vi "FibreSqeezerVI.vi"() -> ()   [LabVIEW 2011]
uses:
  <vilib>/DAQmx/write.llb/DAQmx Write (Analog DBL 1Chan 1Samp).vi
  <vilib>/DAQmx/create/channels.llb/DAQmx Create Channel (AO-Voltage-Basic).vi
  <vilib>/DAQmx/configure/timing.llb/DAQmx Timing (Sample Clock).vi
  <vilib>/DAQmx/miscellaneous.llb/DAQmx Fill In Error Info.vi
  <vilib>/measure/NI_MABase.lvlib
panel:
  in  "frequency":dbl=10.0 format="%0.2p"
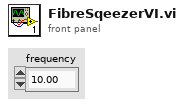
[diagram p1: front panel]
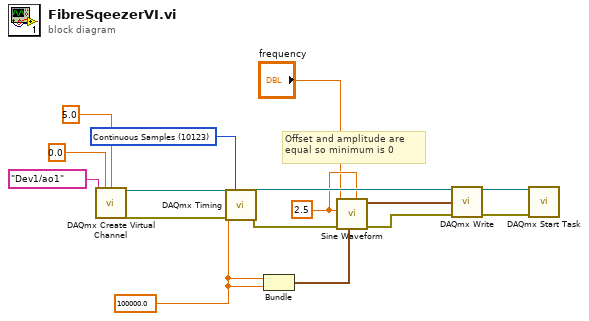
[diagram p0: block diagram]
diagram:
  w4 = 100000.0 ("rate")
  w6 = 2.5 ("amplitude")
  w9 = 10123 items=["Finite Samples"=10178, "Continuous Samples"=10123, "Hardware Timed Single Point"=12522] ("sample mode")
  # "Offset and amplitude are equal so minimum is 0"
  n1 = call-poly <vilib>:"DAQmx Create Virtual Channel.vi"("maximum value"=0.0, "minimum value"=5.0, "physical channels"=tag "Dev1/ao1") -> ("task out"=w15:refnum<k21>, "error out"=w10:errorcluster)  [unwired: 11 in]
  n2 = call-poly <vilib>:"DAQmx Timing.vi"("task/channels in"=w15, "sample mode"=w9, "rate"=w4, "error in"=w10) -> ("task out"=w14:refnum<k21>, "error out"=w11:errorcluster)  [unwired: 10 in]
  n3 = Bundle("rate"=w4, "rate"=w4) -> (w5:cluster{"rate":dbl, "rate":dbl})  [unwired: 1 in]
  n4 = call <vilib>:"Sine Waveform.vi"("offset"=w6, "sampling info"=w5, "error in (no error)"=w11, "amplitude"=w6, "frequency"="frequency") -> ("error out"=w12:errorcluster, "signal out"=w13:waveform(dbl))  [unwired: 5 in]
  n5 = call-poly <vilib>:"DAQmx Write.vi"("task/channels in"=w14, "data"=w13, "error in"=w12) -> ("task out"=w2:refnum<k21>, "error out"=w1:errorcluster)  [unwired: 10 in, 1 out]
  n6 = call <vilib>:"DAQmx Start Task.vi"("task/channels in"=w2, "error in"=w1) -> ()  [unwired: 12 in, 2 out]
